vi "FormatCSVHeader.vi"(4 "Measurement Type":string, 6 "Notes":string, 7 "Temp":dbl, 8 "Test Path":string, 9 "Wirings":string[](array[string]), 10 "Loads":dbl[](array[numeric]), 11 "Voltages":dbl[](array[numeric])=[18.0, 24.0, 36.0]) -> (2 "Output String":string)   [LabVIEW 2013]
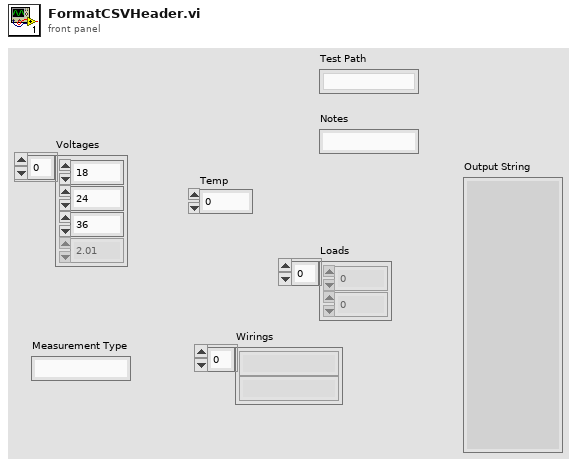
[diagram p1: front panel]
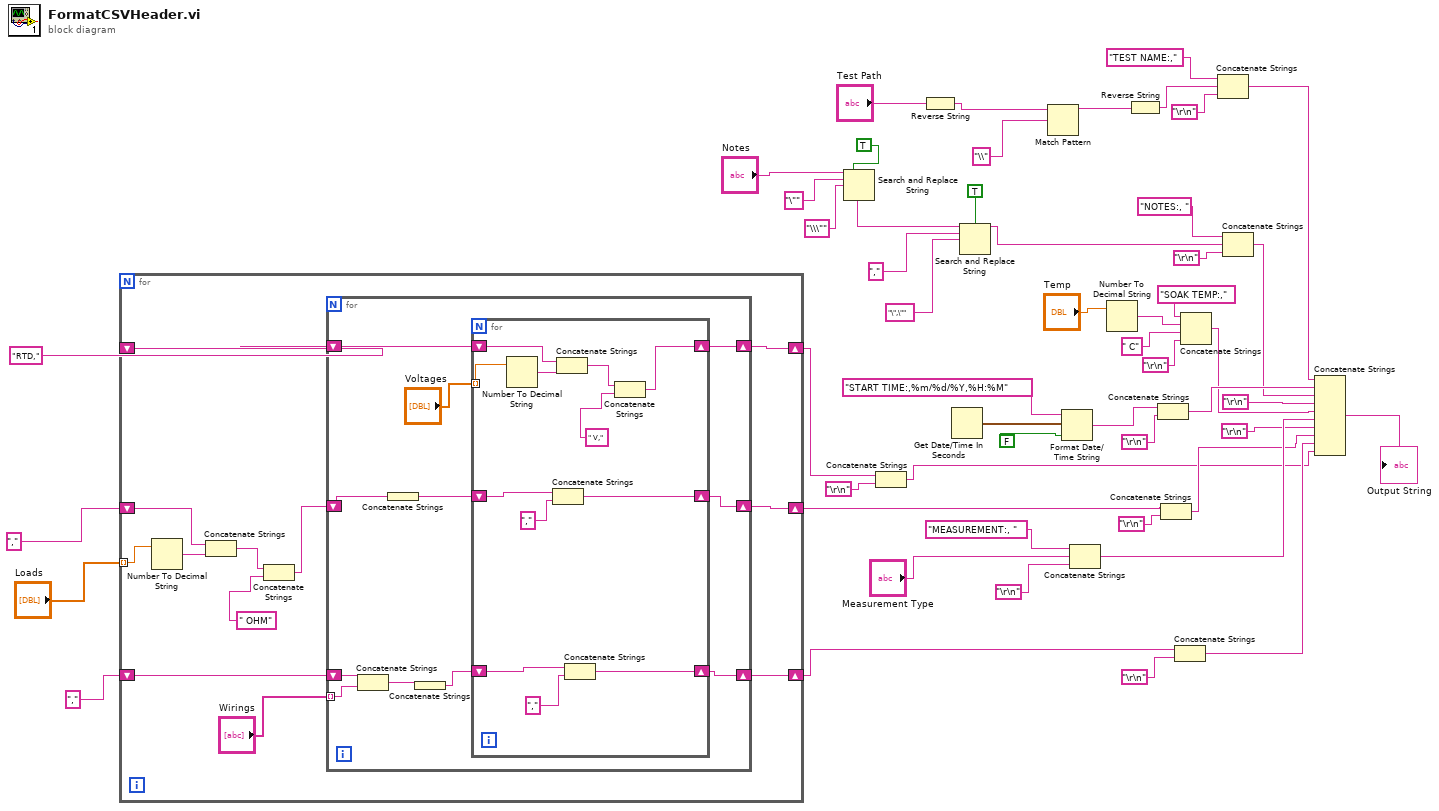
[diagram p0: block diagram]
diagram:
  n1 = for {
    shift-right: [w64] -> w7
    shift-left: "," -> [w57]
    shift-right: [w63] -> w9
    shift-left: "RTD," -> [w62]
    tunnel: "Loads" -> [w58] mode=indexing
    shift-right: [w54] -> w5
    shift-left: "," -> [w53]
    n2 = Number To Decimal String(number=w58) -> (decimal integer string=w60:string)  [unwired: 1 in]
    n3 = Concatenate Strings(w57, w60) -> (w59:string)
    n4 = Concatenate Strings(w59, " OHM") -> (w56:string)
    n5 = for {
      shift-right: [w74] -> w63
      shift-left: w62 -> [w73]
      shift-right: [w75] -> w64
      shift-left: w56 -> [w72]
      tunnel: "Wirings" -> [w67] mode=indexing
      shift-right: [w68] -> w54
      shift-left: w53 -> [w65]
      n6 = Concatenate Strings(w65, w67) -> (w66:string)
      n7 = Concatenate Strings(w72) -> (w71:string)
      n8 = Concatenate Strings(w66) -> (w69:string)
      n9 = for {
        tunnel: "Voltages" -> [w85] mode=indexing
        shift-right: [w83] -> w74
        shift-left: w73 -> [w82]
        shift-right: [w86] -> w75
        shift-left: w71 -> [w79]
        shift-right: [w76] -> w68
        shift-left: w69 -> [w77]
        n10 = Number To Decimal String(number=w85) -> (decimal integer string=w81:string)  [unwired: 1 in]
        n11 = Concatenate Strings(w79, ",") -> (w86:string)
        n12 = Concatenate Strings(w82, w81) -> (w80:string)
        n13 = Concatenate Strings(w77, ",") -> (w76:string)
        n14 = Concatenate Strings(w80, " V,") -> (w83:string)
      }
    }
  }
  n15 = Search and Replace String(replace all?=TRUE, input string="Notes", search string="\"", replace string="\\\"") -> (result string=w29:string)  [unwired: 4 in, 3 out]
  n16 = Concatenate Strings(w9, "\r\n") -> (w1:string)
  n17 = Reverse String(1:"Test Path") -> (0:w39:string)
  n18 = Get Date/Time In Seconds() -> (seconds since 1Jan1904=w44:timestamp)
  n19 = Search and Replace String(replace all?=TRUE, input string=w29, search string=",", replace string="\",\"") -> (result string=w25:string)  [unwired: 4 in, 3 out]
  n20 = Match Pattern(string=w39, regular expression="\\") -> (before substring=w34:string)  [unwired: 1 in, 3 out]
  n21 = Format Date/Time String(time format string (%c)="START TIME:,%m/%d/%Y,%H:%M", seconds (now)=w44, UTC format=FALSE) -> (date/time string=w17:string)
  n22 = Concatenate Strings("MEASUREMENT:, ", "Measurement Type", "\r\n") -> (w11:string)
  n23 = Number To Decimal String(number="Temp") -> (decimal integer string=w42:string)  [unwired: 1 in]
  n24 = Reverse String(1:w34) -> (0:w36:string)
  n25 = Concatenate Strings(w17, "\r\n") -> (w15:string)
  n26 = Concatenate Strings(w7, "\r\n") -> (w3:string)
  n27 = Concatenate Strings(w5, "\r\n") -> (w2:string)
  n28 = Concatenate Strings("SOAK TEMP:,", w42, " C", "\r\n") -> (w12:string)
  n29 = Concatenate Strings("TEST NAME:,", w36, "\r\n") -> (w35:string)
  n30 = Concatenate Strings("NOTES:, ", w25, "\r\n") -> (w14:string)
  n31 = Concatenate Strings(w35, w15, w14, "\r\n", w12, w11, "\r\n", w3, w2, w1) -> (→"Output String":string)
